vi "visio.vi"(11 "Array":T1(array[cluster])) -> (1 "Distance (ft)":dbl(knob) scale=0.0..20.0, 2 "Y":dbl(knob) scale=-20.0..20.0, 3 "X":dbl(knob) scale=-20.0..20.0, 4 "Target Info":T1(array[cluster]))   [LabVIEW 2011]
uses:
  Robot Prototype 2012/Robot Global Data.vi
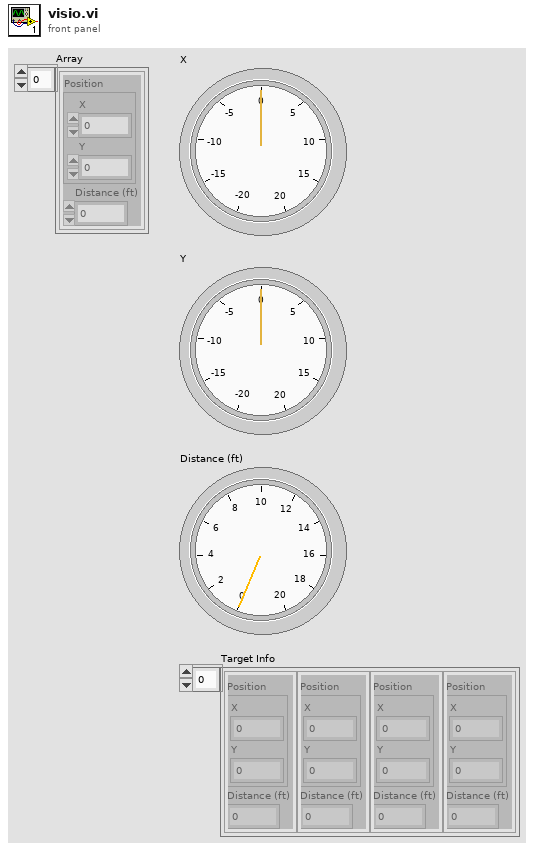
[diagram p1: front panel]
types:
  T1 = cluster{"Position":cluster{"X":dbl, "Y":dbl}, "Distance (ft)":dbl}[]
  T2 = cluster{"Array[0]":cluster{"Position":cluster{"X":dbl, "Y":dbl}, "Distance (ft)":dbl}, "Array[1]":cluster{"Position":cluster{"X":dbl, "Y":dbl}, "Distance (ft)":dbl}, "Array[2]":cluster{"Position":cluster{"X":dbl, "Y":dbl}, "Distance (ft)":dbl}, "Array[3]":cluster{"Position":cluster{"X":dbl, "Y":dbl}, "Distance (ft)":dbl}, "Array[4]":cluster{"Position":cluster{"X":dbl, "Y":dbl}, "Distance (ft)":dbl}, "Array[5]":cluster{"Position":cluster{"X":dbl, "Y":dbl}, "Distance (ft)":dbl}, "Array[6]":cluster{"Position":cluster{"X":dbl, "Y":dbl}, "Distance (ft)":dbl}, "Array[7]":cluster{"Position":cluster{"X":dbl, "Y":dbl}, "Distance (ft)":dbl}, "Array[8]":cluster{"Position":cluster{"X":dbl, "Y":dbl}, "Distance (ft)":dbl}}
  T3 = cluster{"Position":cluster{"X":dbl, "Y":dbl}, "Distance (ft)":dbl}
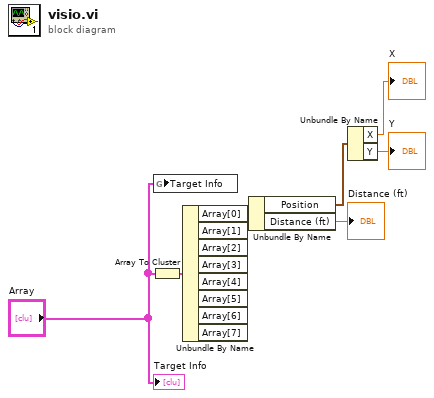
[diagram p0: block diagram]
diagram:
  n1 = Array To Cluster(array="Array") -> (cluster=w7:T2)
  n2 = global write "Robot Global Data.vi" "Target Info"("Array") -> ()
  n3 = Unbundle By Name(w7) -> ("Array[0]"=w2:T3)  [unwired: 7 out]
  n4 = Unbundle By Name(w2) -> ("Position"=w3:cluster{"X":dbl, "Y":dbl}, "Distance (ft)"=→"Distance (ft)":dbl)
  n5 = Unbundle By Name(w3) -> ("X"=→"X":dbl, "Y"=→"Y":dbl)
  "Target Info" <- "Array"
